vi "SetMotors_with_PID.vi"(10 "PID gains":T1(array[cluster])=[{"proportional gain (Kc)"=2.9, "integral time (Ti, min)"=0.002, "derivative time (Td, min)"=0.0}, {"proportional gain (Kc)"=2.9, "integral time (Ti, min)"=0.002, "derivative time (Td, min)"=0.0}, {"proportional gain (Kc)"=2.9, "integral time (Ti, min)"=0.002, "derivative time (Td, min)"=0.0}, {"proportional gain (Kc)"=2.9, "integral time (Ti, min)"=0.002, "derivative time (Td, min)"=0.0}] {"derivative time (Td, min)" format="%.3f"; "integral time (Ti, min)" format="%.3f"; "proportional gain (Kc)" format="%.3f"}, 11 "steering frame velocity":dbl[](array[numeric])=[0.0, 0.0, 0.0]) -> (2 "ccw motor velocity setpoints":dbl[](array[numeric])=[-0.0, -0.0, -0.0, -0.0], 3 "Radians/s":dbl[](array[numeric]))   [LabVIEW 2018]
uses:
  <vilib>/robotics/Steering/Wheel/Wheel Parameters.ctl
  <vilib>/robotics/Steering/Wheel/Rotation Direction.ctl
  <vilib>/robotics/Steering/Omnidirectional Wheel/NI_Robotics_Omnidirectional Wheel.lvclass
  C:/Program Files (x86)/National Instruments/LabVIEW 2018/vi.lib/robotics/Steering/Wheel/NI_Robotics_Wheel.lvclass
  <vilib>/robotics/Steering/Omnidirectional Wheel/Create Omnidirectional Wheel.vi
  <vilib>/robotics/Steering/Steering Frame/Create User Defined Steering Frame.vi
  <vilib>/robotics/Steering/Steering Frame/Apply Steering Frame Velocity to Motors.vi
  <vilib>/addons/control/pid/pid.llb/PID (DBL Array).vi
  <vilib>/robotics/Steering/Create Steering Frame/NI_Robotics_Create Steering Frame.xnode
  <vilib>/robotics/Steering/Class Type Definitions/Steering Frame.ctl
  <vilib>/robotics/Steering/Steering Frame/NI_Robotics_Steering Frame.lvclass
  <vilib>/addons/control/pid/NI_PID_pid.lvlib
  <vilib>/robotics/Steering/Class Type Definitions/NI_Robotics_Steering Class Types.lvlib
  <vilib>/robotics/Steering/Wheel/NI_Robotics_Wheel.lvclass
panel:
  in  "Reset Encoders":bool
  out "Oikea":cluster{"initial PV":dbl, "SP:":dbl}(graph)={"initial PV"=0.0, "SP:"=-0.0}
  out "Vasen":cluster{"initial PV":dbl, "SP:":dbl}(graph)={"initial PV"=0.0, "SP:"=-0.0}
  out "Taka":cluster{"initial PV":dbl, "SP:":dbl}(graph)={"initial PV"=0.0, "SP:"=-0.0}
  out "Etu":cluster{"initial PV":dbl, "SP:":dbl}(graph)={"initial PV"=0.0, "SP:"=-0.0}
  # "Etu"
  # "Taka"
  # "Vasen"
  # "Oikea"
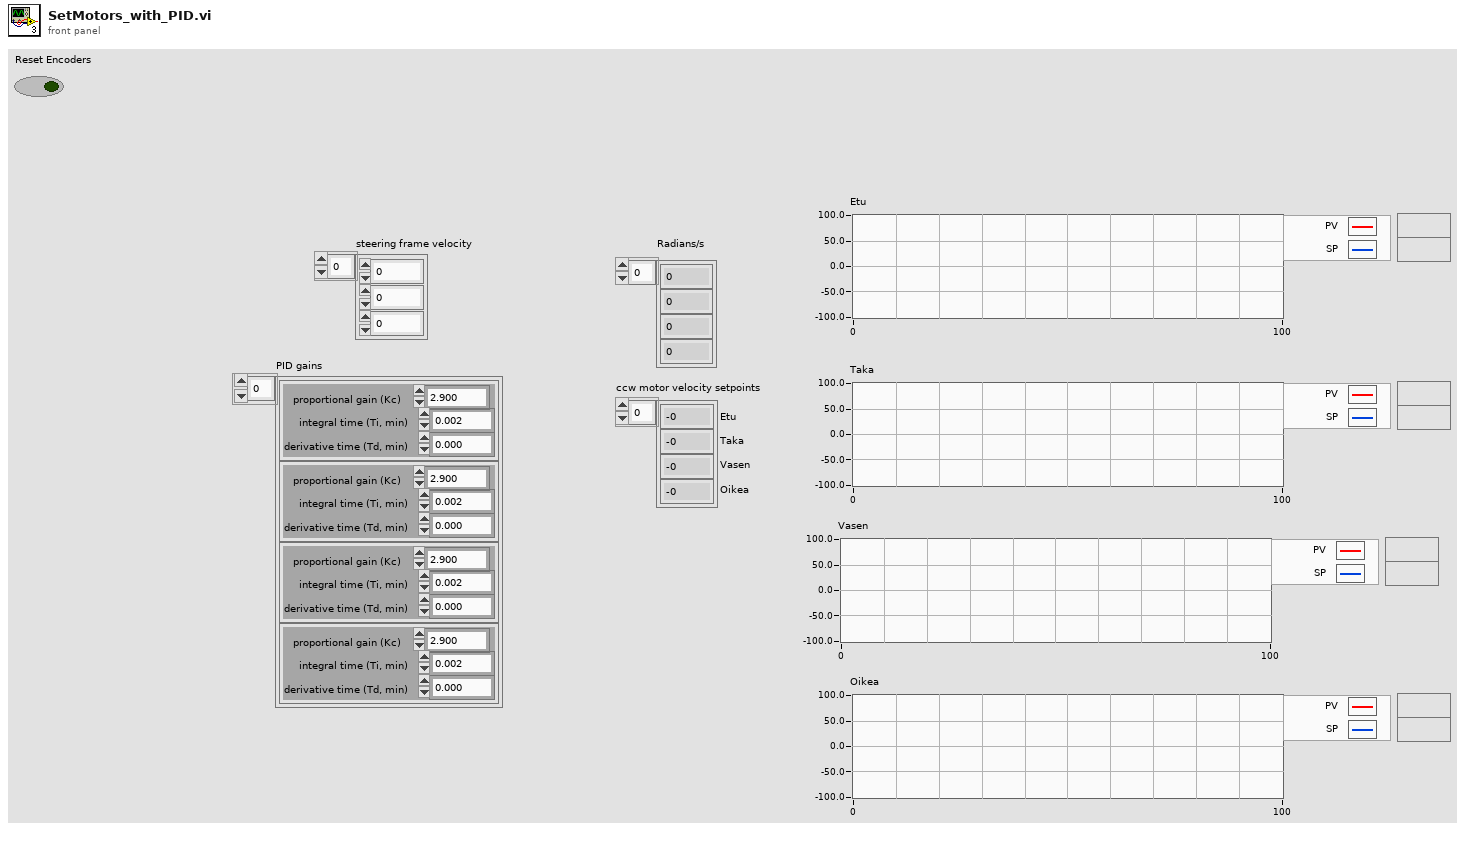
[diagram p1: front panel]
types:
  T1 = cluster{"proportional gain (Kc)":dbl, "integral time (Ti, min)":dbl, "derivative time (Td, min)":dbl}[]
  T2 = cluster{bool, "Tick Count(uSec)":u32, "Counter Value":i32[], "x-y":i32[]}
  T3 = typedef "NI_Robotics_Steering Class Types.lvlib/Steering Frame.ctl" = refnum<class "NI_Robotics_Steering Frame.lvclass">
  T4 = cluster{"Position":i32[], "Velocity RPM":dbl[], "Velocity RPS":dbl[], "Radians/s":dbl[]}
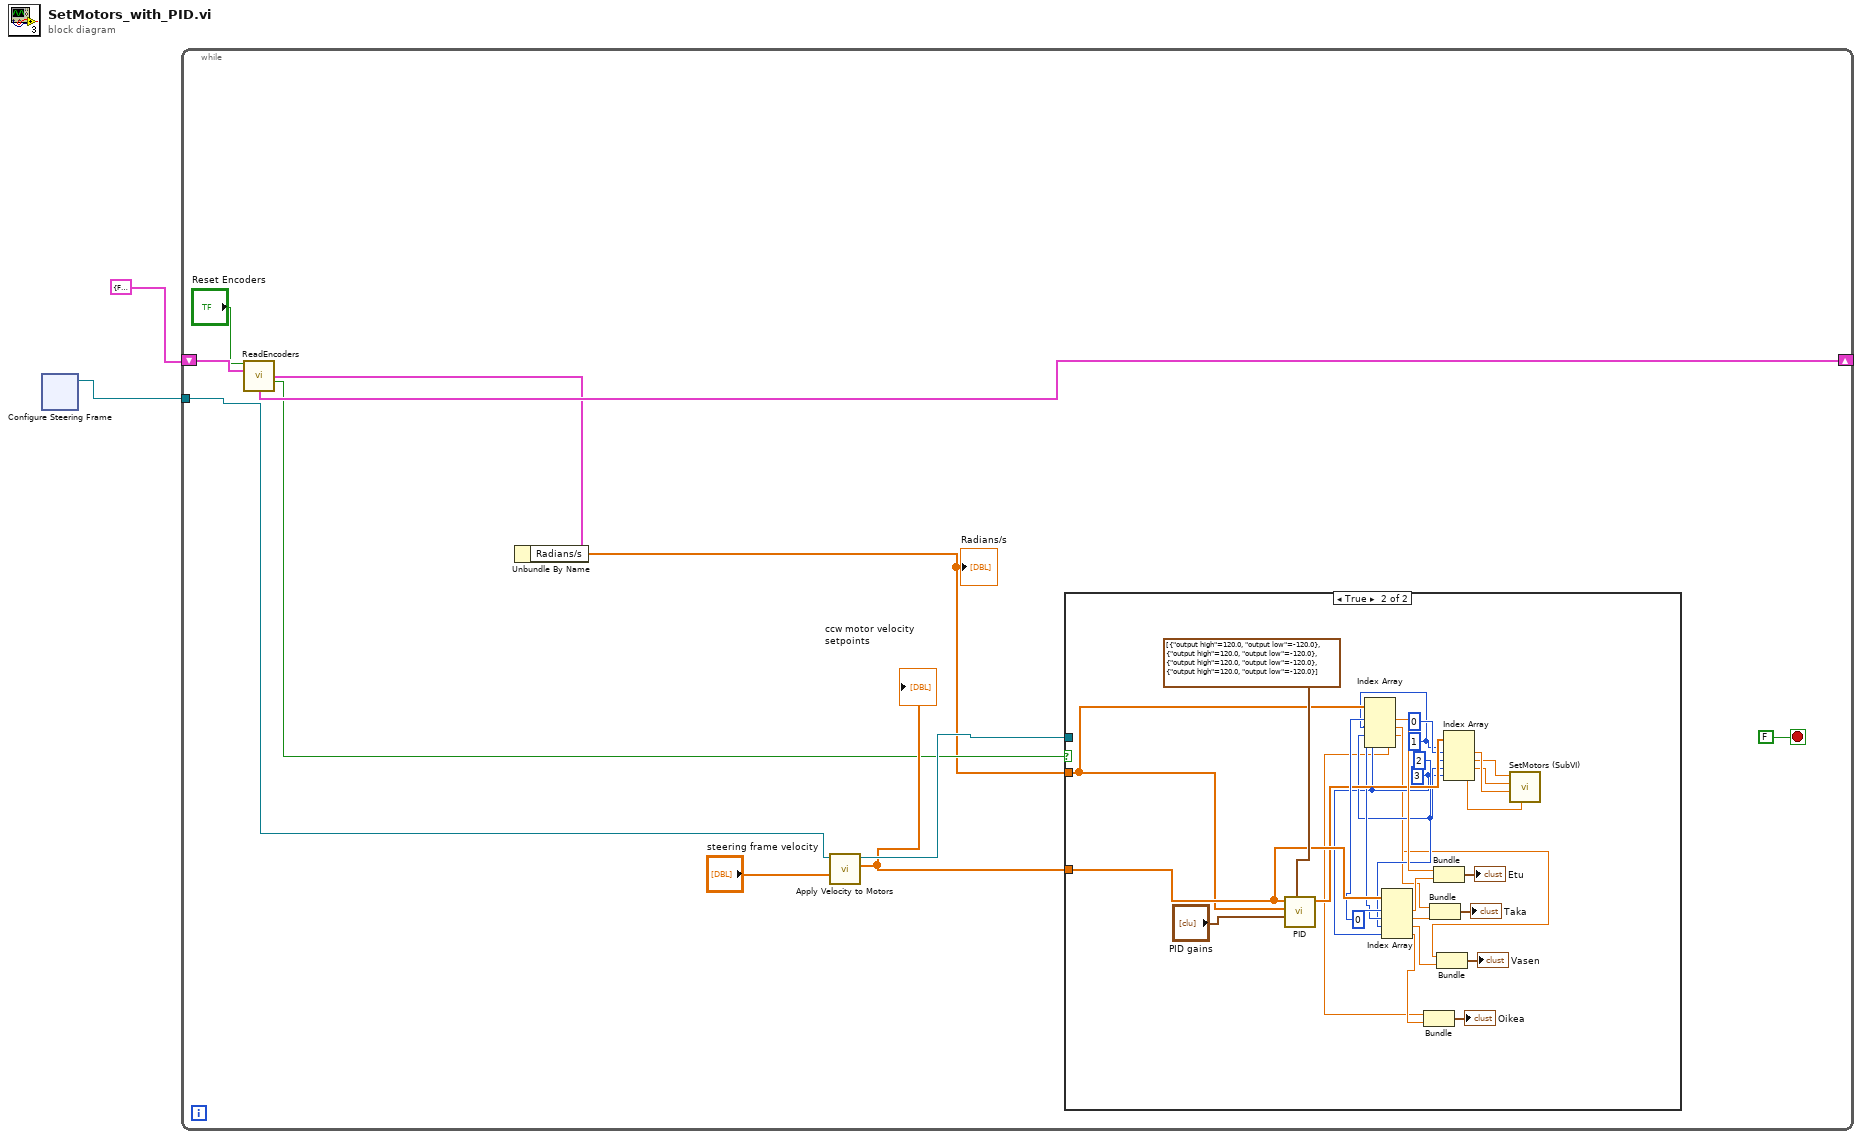
[diagram p0: block diagram]
diagram:
  n1 = xnode ("Configure Steering Frame")() -> ("steering frame out"=w2:T3)  [unwired: 1 in, 1 out]
  n2 = while {
    shift-right: [w8] -> _
    shift-left: T2 {FALSE, "Tick Count(uSec)"=0, "Counter Value"=[0, 0, 0, 0], "x-y"=[0, 0, 0, 0]} ("Cluster in") -> [w5]
    tunnel: w2 -> [w12]
    stop <- FALSE stop-if-true
    n3 = call "ReadEncoders.vi"("Reset Encoders"="Reset Encoders", "Cluster in"=w5) -> ("output cluster"=w7:T4, "Cluster Out"=w8:T2, "Updated"=w6:bool)  [unwired: 9 in, 2 out]
    n4 = Unbundle By Name(w7) -> ("Radians/s"=w4:dbl[])
    "Radians/s" <- w4
    n5 = call-poly <vilib>:"Apply Velocity to Motors.vi"("steering frame velocity"="steering frame velocity", "steering frame in"=w12) -> ("ccw motor velocity setpoints"=w9:dbl[], "steering frame out"=w11:T3)  [unwired: 5 in, 3 out]
    "ccw motor velocity setpoints" <- w9
    n6 = case shown="True" w6 {
      tunnel: w11 -> [_ _]
      tunnel: w9 -> [_ w37]
      tunnel: w4 -> [_ w32]
      frame False {
      }
      frame True {
        w17 = 3 ("index")
        w18 = 2 ("index")
        w19 = 1 ("index")
        w36 = 0 ("index")
        n7 = call-poly <vilib>:"PID.vi"("output range"=cluster{"output high":dbl, "output low":dbl}[] [{"output high"=120.0, "output low"=-120.0}, {"output high"=120.0, "output low"=-120.0}, {"output high"=120.0, "output low"=-120.0}, {"output high"=120.0, "output low"=-120.0}], "PID gains"="PID gains", "process variable"=w32, "setpoint"=w37) -> ("output"=w31:dbl[])  [unwired: 6 in, 1 out]
        n8 = Index Array(array=w32, index #1=w36, index #2=w19, index #3=w18, index #4=w17) -> (element #1=w34:dbl, element #2=w16:dbl, element #3=w15:dbl, element #4=w14:dbl)
        n9 = Index Array(array=w37, index #1=w36, index #2=w19, index #3=w18, index #4=w17) -> (element #1=w33:dbl, element #2=w20:dbl, element #3=w21:dbl, element #4=w22:dbl)
        n10 = Bundle(w14, "Numeric"=w22) -> (→"Oikea":cluster{dbl, "Numeric":dbl})  [unwired: 1 in]
        n11 = Bundle(w16, "Numeric"=w20) -> (→"Taka":cluster{dbl, "Numeric":dbl})  [unwired: 1 in]
        n12 = Bundle(w34, "Numeric"=w33) -> (→"Etu":cluster{dbl, "Numeric":dbl})  [unwired: 1 in]
        n13 = Bundle(w15, "Numeric"=w21) -> (→"Vasen":cluster{dbl, "Numeric":dbl})  [unwired: 1 in]
        n14 = Index Array(array=w31, index #1=0 ("index"), index #2=w19, index #3=w18, index #4=w17) -> (element #1=w29:dbl, element #2=w28:dbl, element #3=w27:dbl, element #4=w26:dbl)
        n15 = call "SetMotors (SubVI).vi"("Oikea"=w26, "Etu"=w29, "Vasen"=w27, "Taka"=w28) -> ()  [unwired: 8 in]
      }
    }
  }
